vi "AfterPage2_UI.vi"(10 "MetaDataObj":refnum<class "MetaDataObj.lvclass">) -> ()   [LabVIEW 2021, in "CIF_Plugin_Generator.lvclass"]
uses:
  CIF_Plugin_Generator.lvclass
  <resource>/dialog/NewProjectWizard/MetaDataObj/MetaDataObj.lvclass
  C:/Program Files/National Instruments/LabVIEW 2021/resource/dialog/NewProjectWizard/MetaDataObj/MetaDataObj.lvclass
  <resource>/dialog/NewProjectWizard/MetaDataObj/MetaDataObj.lvclass/MetaDataObj.ctl
  CIF_Plugin_Generator.lvclass/CIF_Plugin_Generator.ctl
  2b3e1c27-d443-4546-a5b6-192e9e090b09.vi
  <resource>/dialog/NewProjectWizard/MetaDataObj/Accessors/Read Project Root.vi
  <resource>/dialog/NewProjectWizard/MetaDataObj/Accessors/Read Project Name.vi
  <resource>/dialog/NewProjectWizard/MetaDataObj/Accessors/Read Overlay Pixmap.vi
  <vilib>/LabVIEW Icon API/lv_icon/Classes/Icon/Icon.lvclass
  Plugin Generator.lvlib
  <vilib>/CIF Foundation/CIF Utilities/Errors/Errors_CIF_U.lvlib
panel:
  out "To display":string
  out "Plugin Generation Status":string
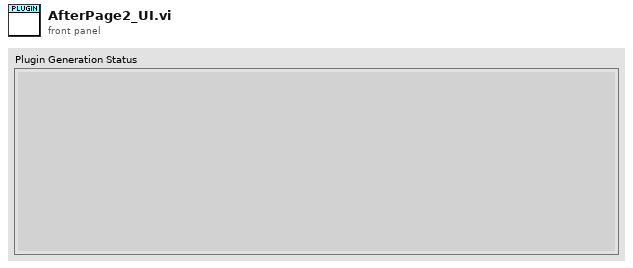
[diagram p1: front panel]
types:
  T1 = typedef "ChannelRegistrar.lvlib/Channel Definition for Scripting.ctl" = cluster{"Name":string, "Direction":T2, "Type":T3}
  T2 = typedef "CIFChannels.lvclass/Direction.ctl" = enum16{"Publisher", "Subscriber"}
  T3 = typedef "ChannelRegistrar.lvlib/Registered Channel Types.ctl" = enum16{"Custom", "Double_Tag", "I64_Tag", "U64_Tag", "U8_FIFO", "CAN_FIFO", "L2Enet_FIFO", "DAQ_FIFO", "Universal_FIFO", "String_Tag"}
  T4 = typedef "Plugin Generator.lvlib/Documentation Info.ctl" = cluster{"Description":string, "Author":string}
  T5 = typedef "Plugin Generator.lvlib/Proto Names.ctl" = cluster{"PascalCase":string, "snake_case":string}
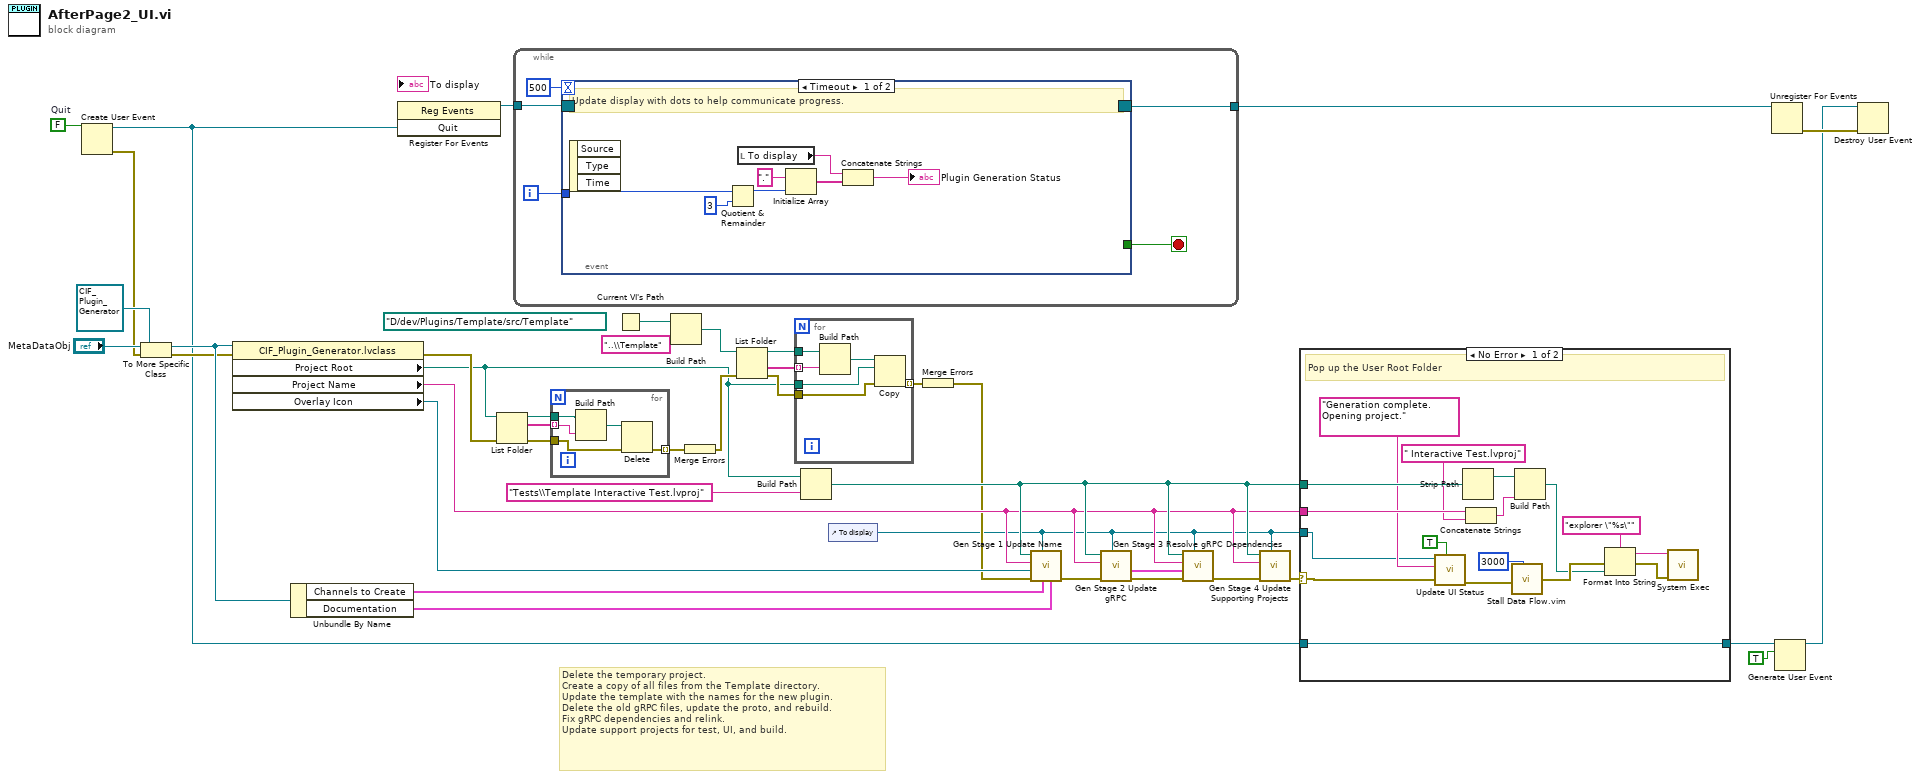
[diagram p0: block diagram]
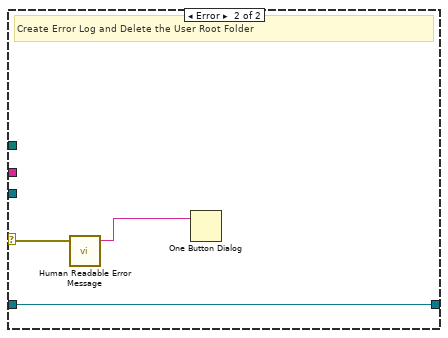
[diagram p2: hidden frame]
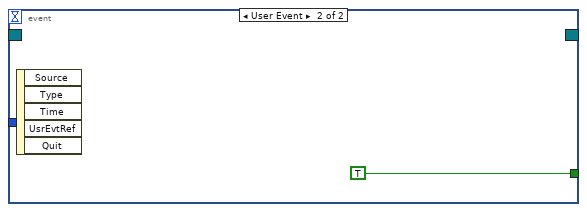
[diagram p3: hidden frame]
diagram:
  w23 = FALSE  # Quit
  (unwired) path "D:/dev/Plugins/Template/src/Template" ("source path")
  # "Delete the temporary project.\nCreate a copy of all files from the Template directory.\nUpdate the template with the names for the new plugin.\nDelete the old gRPC files, update the proto, and rebuild.\nFix gRPC dependencies and relink.\nUpdate support projects for test, UI, and build."
  n1 = Create User Event(user event datatype=w23) -> (user event=w16:refnum<user-event>, error out=w15:errorcluster)  [unwired: 1 in]
  n2 = To More Specific Class(target class=refnum<class "CIF_Plugin_Generator.lvclass"> refnum ("Plugin_Generator.lvclass"), reference="MetaDataObj", error in=w15) -> (specific class reference=w39:refnum<class "CIF_Plugin_Generator.lvclass">, error out=w38:errorcluster)
  n3 = property class="CIF_Plugin_Generator.lvclass"(reference=w39, error in=w38) -> (error out=w33:errorcluster, "Project Root"=w27:path, "Project Name"=w10:string, "Overlay Icon"=w25:refnum<class "Icon.lvclass">)  [unwired: 1 out]
  n4 = Unbundle By Name(w39) -> ("Channels to Create"=w24:T1[], "Documentation"=w4:T4)
  n5 = register-events(w16) -> (reference out=w22:refnum<event-registration>)  [unwired: 2 in, 1 out]
  n6 = List Folder(path=w27, error in=w33) -> (path out=w36:path, filenames=w35:string[], error out=w34:errorcluster)  [unwired: 2 in, 1 out]
  n7 = while {
    tunnel: w22 -> [w44]
    tunnel: [w41] -> w20
    i -> [w42]
    stop <- w43 stop-if-true
    n8 = event shown="[0] Timeout" {
      selector: w44 -> [_ _]
      dyn-events: [_ _] -> w41
      timeout: 500 -> [_ _]
      tunnel: [_ TRUE] -> w43
      tunnel: w42 -> [w52 _]
      event Timeout {
        # "Update display with dots to help communicate progress."
        n9 = event-data() -> ()  [unwired: 1 in, 3 out]
        n10 = Quotient & Remainder(x=w52, y=3) -> (x-y*floor(x/y)=w50:i32)  [unwired: 1 out]
        n11 = local read "To display"() -> (w51:string)
        n12 = Initialize Array(".", w50) -> (w48:string[])
        n13 = Concatenate Strings(w51, w48) -> (→"Plugin Generation Status":string)
      }
      event User Event {
        n14 = event-data() -> ()  [unwired: 1 in, 5 out]
      }
    }
  }
  n15 = for {
    tunnel: w36 -> [w58]
    tunnel: w35 -> [w57] mode=indexing
    tunnel: w34 -> [w55]
    tunnel: [w54] -> w32 mode=indexing
    n16 = Build Path(base path=w58, name or relative path=w57) -> (appended path=w56:path)
    n17 = Delete(path (use dialog)=w56, error in=w55) -> (error out=w54:errorcluster)  [unwired: 3 in, 2 out]
  }
  n18 = Current VI's Path() -> (path=w3:path)
  n19 = Build Path(base path=w3, name or relative path="..\\Template") -> (appended path=w1:path)
  n20 = Merge Errors(w32) -> (w29:errorcluster)
  n21 = List Folder(path=w1, error in=w29) -> (path out=w31:path, folder names=w30:string[], error out=w28:errorcluster)  [unwired: 2 in, 1 out]
  n22 = for {
    tunnel: w31 -> [w64]
    tunnel: w28 -> [w62]
    tunnel: w30 -> [w63] mode=indexing
    tunnel: w27 -> [w60]
    tunnel: [w59] -> w13 mode=indexing
    n23 = Build Path(base path=w64, name or relative path=w63) -> (appended path=w61:path)
    n24 = Copy(8:w62, 10:w60, 11:w61) -> (0:w59:errorcluster)  [unwired: 2 in, 2 out]
  }
  n25 = Build Path(base path=w27, name or relative path="Tests\\Template Interactive Test.lvproj") -> (appended path=w11:path)
  n26 = control-ref of="To display"() -> (w5:refnum<vi>)
  n27 = Merge Errors(w13) -> (w9:errorcluster)
  n28 = call "Gen Stage 1 Update Name.vi"("Documentation"=w4, "Channels to Create"=w24, "Staus"=w5, "error in"=w9, "Overlay Icon"=w25, "New Subname"=w10, "Template Project Path"=w11) -> ("error out"=w8:errorcluster)  [unwired: 4 in]
  n29 = call "Gen Stage 2 Update gRPC.vi"("Staus"=w5, "error in"=w8, "New Subname"=w10, "Template Project Path"=w11) -> ("error out"=w7:errorcluster, "Proto Names"=w12:T5)  [unwired: 6 in]
  n30 = call "Gen Stage 3 Resolve gRPC Dependencies.vi"("Staus"=w5, "error in"=w7, "Proto Names"=w12, "New Subname"=w10, "Template Project Path"=w11) -> ("error out"=w6:errorcluster)  [unwired: 6 in]
  n31 = call "Gen Stage 4 Update Supporting Projects.vi"("Staus"=w5, "error in (no error)"=w6, "New Name"=w10, "Template Project Path"=w11) -> ("error out"=w14:errorcluster)  [unwired: 7 in]
  n32 = case shown="No Error" w14 {
    selector: w14 -> [w66 w83]
    tunnel: [w78 w84] -> w17
    tunnel: w16 -> [w78 w84]
    tunnel: w11 -> [w75 _]
    tunnel: w10 -> [w71 _]
    tunnel: w5 -> [w67 _]
    frame No Error {
      # "Pop up the User Root Folder"
      n33 = call "Update UI Status.vi"("Previous Complete"=TRUE, "error in"=w66, "Status to Display"="Generation complete.  Opening project." ("To display"), "String in"=w67) -> ("error out"=w65:errorcluster)  [unwired: 7 in]
      n34 = Strip Path(path=w75) -> (stripped path=w74:path)  [unwired: 1 out]
      n35 = Concatenate Strings(w71, " Interactive Test.lvproj" ("string")) -> (w72:string)
      n36 = call "Stall Data Flow.vim"("value in"=w65, "milliseconds to wait"=u32 3000) -> ("value out"=w77:errorcluster)  [unwired: 1 out]
      n37 = Build Path(base path=w74, name or relative path=w72) -> (appended path=w73:path)
      n38 = Format Into String(format string="explorer \"%s\"", error in=w77, w73) -> (resulting string=w81:string, error out=w79:errorcluster)  [unwired: 1 in]
      n39 = call <vilib>:"System Exec.vi"("error in (no error)"=w79, "command line"=w81) -> ()  [unwired: 6 in, 4 out]
    }
    frame Error {
      # "Create Error Log and Delete the User Root Folder"
      n40 = call <vilib>:"Human Readable Error Message.vi"("error in (no error)"=w83) -> ("Human readable error message"=w82:string)  [unwired: 4 in]
      n41 = One Button Dialog(message=w82) -> ()  [unwired: 1 in, 1 out]
    }
  }
  n42 = Unregister For Events(event registration refnum=w20) -> (error out=w19:errorcluster)  [unwired: 1 in]
  n43 = Generate User Event(user event=w17, event data cluster=TRUE ("event data")) -> (user event out=w18:refnum<user-event>)  [unwired: 2 in, 1 out]
  n44 = Destroy User Event(user event=w18, error in=w19) -> ()  [unwired: 1 out]
